vi "Close.vi"(8 "error in":errorcluster, 11 "4-20mA Out Settings In":T1) -> (0 "error out":errorcluster, 3 "4-20mA Out Settings Out":T1)   [LabVIEW 2018, in "Pressure Regulator Library.lvlib"]
uses:
  Pressure Regulator Library.lvlib
  Pressure Regulator Device Settings.ctl
  <vilib>/DAQmx/write.llb/DAQmx Write (Analog DBL 1Chan 1Samp).vi
  <vilib>/DAQmx/miscellaneous.llb/DAQmx Fill In Error Info.vi
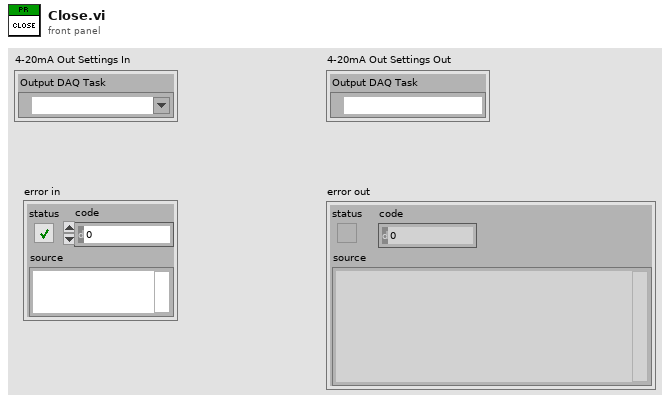
[diagram p1: front panel]
types:
  T1 = typedef "Pressure Regulator Library.lvlib/Pressure Regulator Device Settings.ctl" = cluster{"Output DAQ Task":refnum<k21>}
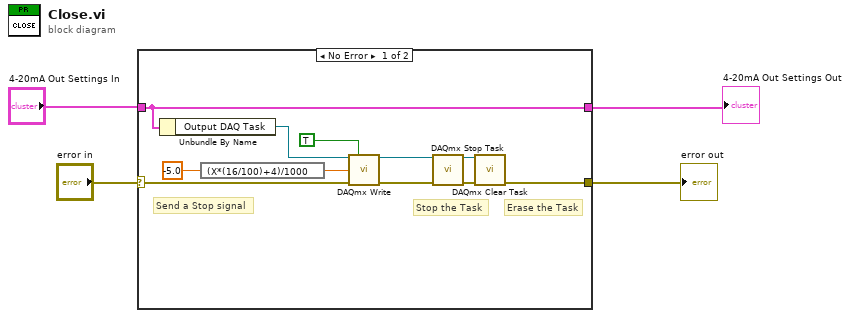
[diagram p0: block diagram]
diagram:
  n1 = case shown="No Error" "error in" {
    selector: "error in" -> [w10 w17]
    tunnel: [w13 w17] -> w3
    tunnel: "4-20mA Out Settings In" -> [w7 w16]
    tunnel: [w7 w16] -> w2
    frame No Error {
      # "Erase the Task"
      # "Stop the Task"
      # "Send a Stop signal"
      n2 = Unbundle By Name(w7) -> ("Output DAQ Task"=w9:refnum<k21>)
      n3 = expression code="(X*(16/100)+4)/1000"(-5.0 ("data")) -> (w5:dbl)
      n4 = call-poly <vilib>:"DAQmx Write.vi"("task/channels in"=w9, "auto start"=TRUE, "data"=w5, "error in"=w10) -> ("task out"=w8:refnum<k21>, "error out"=w11:errorcluster)  [unwired: 9 in, 1 out]
      n5 = call <vilib>:"DAQmx Stop Task.vi"("task/channels in"=w8, "error in"=w11) -> ("task out"=w15:refnum<k21>, "error out"=w14:errorcluster)  [unwired: 12 in]
      n6 = call <vilib>:"DAQmx Clear Task.vi"("task in"=w15, "error in"=w14) -> ("error out"=w13:errorcluster)  [unwired: 13 in]
    }
    frame Error {
    }
  }
  "error out" <- w3
  "4-20mA Out Settings Out" <- w2
